vi "Caracterización de mototres por respuesta y constante de tiempo.vi"() -> ()   [LabVIEW 2024]
uses:
  <vilib>/Utility/NIReport.llb/Report Type.ctl
  <vilib>/Instr/_visa.llb/VISA Configure Serial Port (Instr).vi
  <vilib>/addons/_office/excel.llb/Excel Easy Table (str).vi
  <vilib>/Utility/NIReport.llb/NI_report.lvclass
  <vilib>/addons/_office/NI_ReportGenerationToolkit.lvlib
  <vilib>/Utility/NIReport.llb/NI_ReportGenerationCore.lvlib
  <vilib>/Utility/NIReport.llb/Excel/NI_Excel.lvclass
panel:
  in  "template (empty)":path
  out "XY Graph":cluster{"Y":dbl[], "Y":dbl[]}[](graph)
  out "Tiempo":string
  out "Velocidad":string
  out "read buffer":string
  in  "stop":bool
  in  "baud rate (9600)":u32=9600
  in  "VISA resource name":refnum<visa-resource-name>
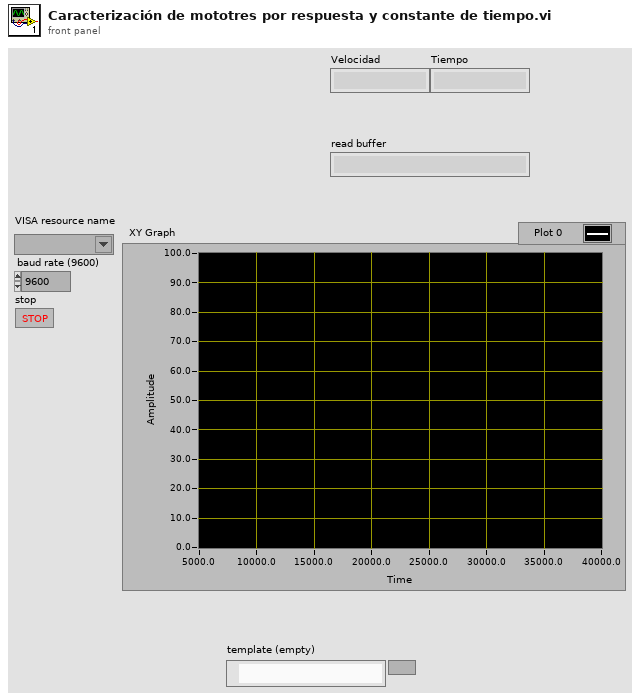
[diagram p1: front panel]
types:
  T1 = typedef "NI_ReportGenerationCore.lvlib/Report Type.ctl" = enum16{"HTML", "Word", "Excel"}
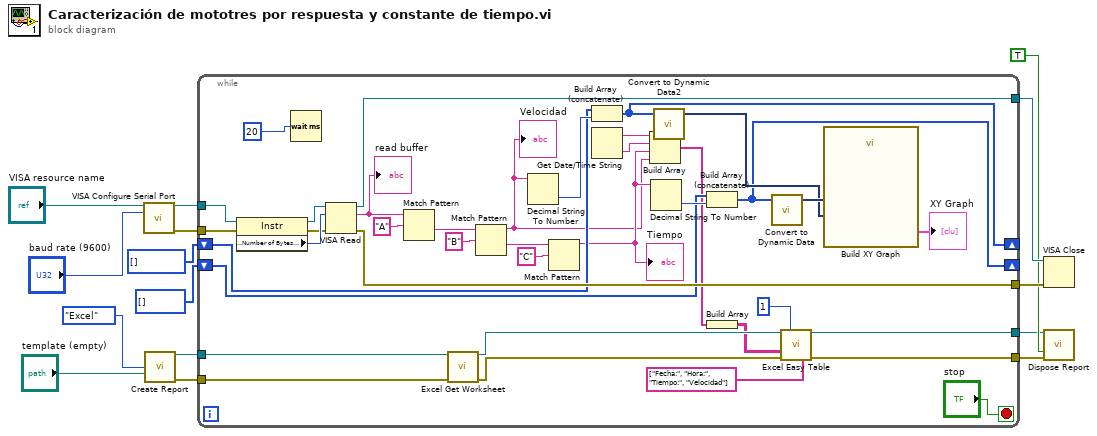
[diagram p0: block diagram]
diagram:
  n1 = call-poly "VISA Configure Serial Port"("VISA resource name"="VISA resource name", "baud rate (9600)"="baud rate (9600)") -> ("VISA resource name out"=w15:refnum<visa-resource-name>, "error out"=w14:errorcluster)  [unwired: 12 in]
  n2 = call <vilib>:"Create Report.vi"("report type"=Report_Type."Excel", "template (empty)"="template (empty)") -> ("report out"=w4:refnum<class "NI_report.lvclass">, "error out"=w3:errorcluster)  [unwired: 12 in]
  n3 = while {
    tunnel: w15 -> [w52]
    tunnel: w14 -> [w49]
    tunnel: [w47] -> w11
    tunnel: [w42] -> w10
    shift-right: [w33] -> _
    shift-left: i32[] [] -> [w31]
    shift-right: [w34] -> _
    shift-left: i32[] [] ("Array") -> [w35]
    tunnel: w4 -> [w23]
    tunnel: w3 -> [w22]
    tunnel: [w20] -> w2
    tunnel: [w19] -> w1
    stop <- "stop" stop-if-true
    n4 = property class="Instr"(reference=w52, error in=w49) -> (reference out=w51:refnum<visa-resource-name>, error out=w48:errorcluster, "Serial Settings:Number of Bytes at Serial Port"=w50:u32)
    n5 = Wait (ms)(milliseconds to wait=u32 20 ("millisecond multiple")) -> ()  [unwired: 1 out]
    n6 = VISA Read(VISA resource name=w51, byte count=w50, error in (no error)=w48) -> (VISA resource name out=w47:refnum<visa-resource-name>, read buffer=w46:string, error out=w42:errorcluster)  [unwired: 1 out]
    "read buffer" <- w46
    n7 = Match Pattern(string=w46, regular expression="A") -> (after substring=w41:string)  [unwired: 1 in, 3 out]
    n8 = call <vilib>:"Excel Get Worksheet.vi"("report in"=w23, "error in (no error)"=w22) -> ("report out"=w24:refnum<class "NI_report.lvclass">, "error out"=w25:errorcluster)  [unwired: 12 in]
    n9 = Match Pattern(string=w41, regular expression="B") -> (before substring=w27:string, after substring=w40:string)  [unwired: 1 in, 2 out]
    "Velocidad" <- w27
    n10 = Decimal String To Number(string=w27) -> (number=w32:i32)  [unwired: 2 in, 1 out]
    n11 = Match Pattern(string=w40, regular expression="C") -> (before substring=w28:string)  [unwired: 1 in, 3 out]
    "Tiempo" <- w28
    n12 = Build Array (concatenate)(w31, w32) -> (w33:i32[])
    n13 = Get Date/Time String() -> (date string=w30:string, time string=w29:string)  [unwired: 3 in]
    n14 = Build Array(w30, w29, w28, w27) -> (w26:string[])
    n15 = Decimal String To Number(string=w28) -> (number=w36:i32)  [unwired: 2 in, 1 out]
    n16 = call "Convert to Dynamic Data2"("Array"=w33) -> ("Dynamic Data Type"=w37:dynamicdata)  [unwired: 3 in]
    n17 = Build Array (concatenate)(w35, w36) -> (w34:i32[])
    n18 = Build Array(w26) -> (w21:string[][])
    n19 = call "Convert to Dynamic Data"("Array"=w34) -> ("Dynamic Data Type"=w38:dynamicdata)  [unwired: 3 in]
    n20 = call-poly <vilib>:"Excel Easy Table.vi"("report in"=w24, "iteration"=1, "text data"=w21, "error in (no error)"=w25, "column headers"=string[] ["Fecha:", "Hora:", "Tiempo:", "Velocidad"]) -> ("report out"=w20:refnum<class "NI_report.lvclass">, "error out"=w19:errorcluster)  [unwired: 6 in, 3 out]
    n21 = call "Build XY Graph"("Y Input"=w37, "X Input"=w38) -> ("XY Graph"=→"XY Graph":cluster{"X":dbl[], "Y":dbl[]}[])  [unwired: 8 in, 1 out]
  }
  n22 = VISA Close(VISA resource name=w11, error in (no error)=w10) -> ()  [unwired: 1 out]
  n23 = call-dynamic "Dispose Report.vi"("report in"=w2, "save changes? (F)"=TRUE, "error in (no error)"=w1) -> ()  [unwired: 12 in, 1 out]
